vi "WPI_CameraSend Images To PC Loop.vi"(8 "error in (no error)":errorcluster, 9 "port":u16=1181) -> ()   [LabVIEW 2017]
doc: "This VI is used to serve images from one or more named cameras on your robot to the dashboard, SmartDashboard, or compatible web browser. Camera name and type info is published using network tables. Connections are on port 1181 by default and the URL for streaming can be found by looking at the network \"camera\"/streams variable. Cameras that are opened and stored in the name registry are automatically published by that name.\n\nThis VI runs in parallel with other code and should be placed in Robot Main or in Periodic Tasks.\n\nThis software is licensed. Open the labview\\readme\\WPI Robotics Library Open Source License.txt file for more information."
uses:
  <vilib>/Rock Robotics/WPI/Utilities/Refnum Registry Operation.ctl
  <vilib>/Rock Robotics/Network Tables/NT Write String Array.vi
  <vilib>/Rock Robotics/Network Tables/NT Write String.vi
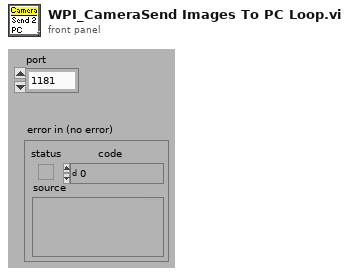
[diagram p1: front panel]
types:
  T1 = enum16{"Standard", "Buffered", "CRLF", "Immediate"}
  T2 = typedef "Refnum Registry Operation.ctl" = enum16{"set", "get", "delete", "get all names", "read name"}
  T3 = cluster{"token string":string, "token string 2":string}[]
  T4 = typedef "WPI_CameraDevRef.ctl" = cluster{"Camera Address":string, "CameraStatus":errorcluster}
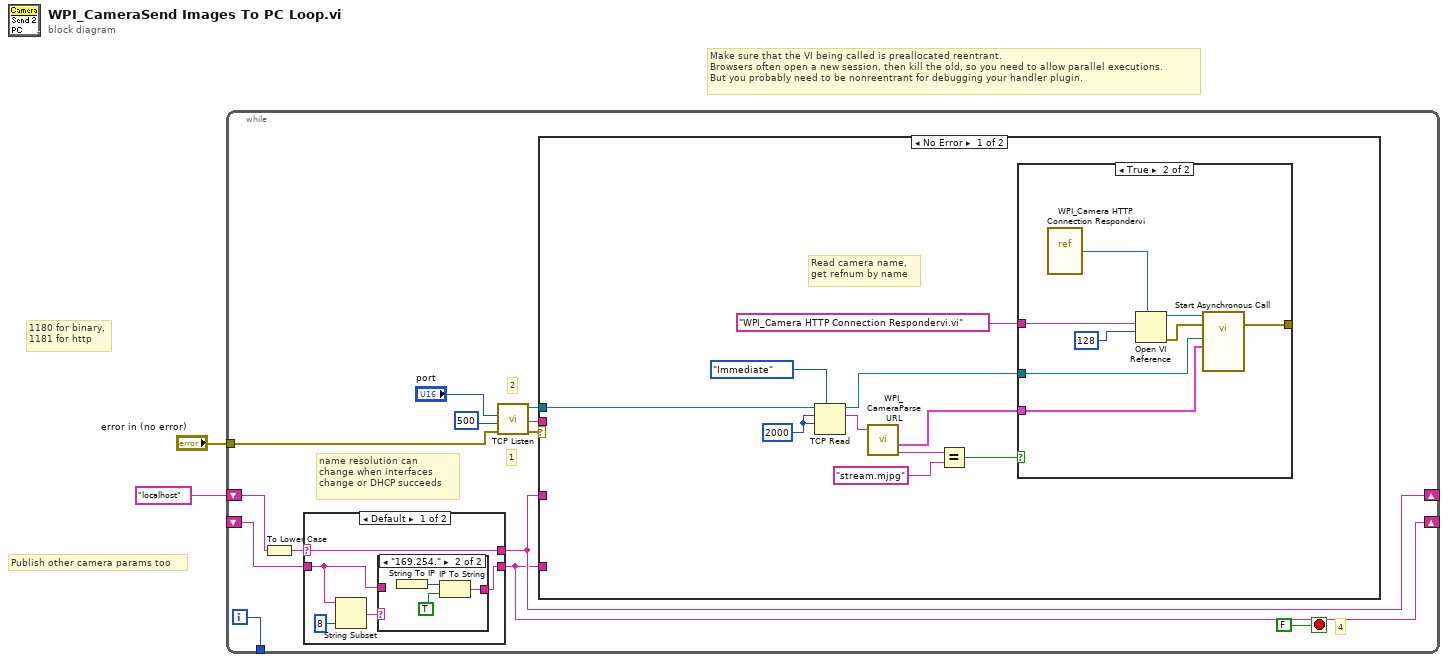
[diagram p0: block diagram]
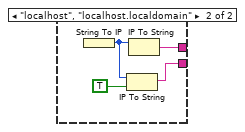
[diagram p3: hidden frame]
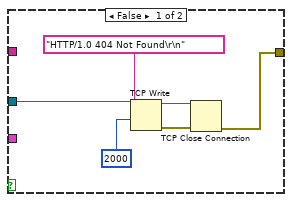
[diagram p4: hidden frame]
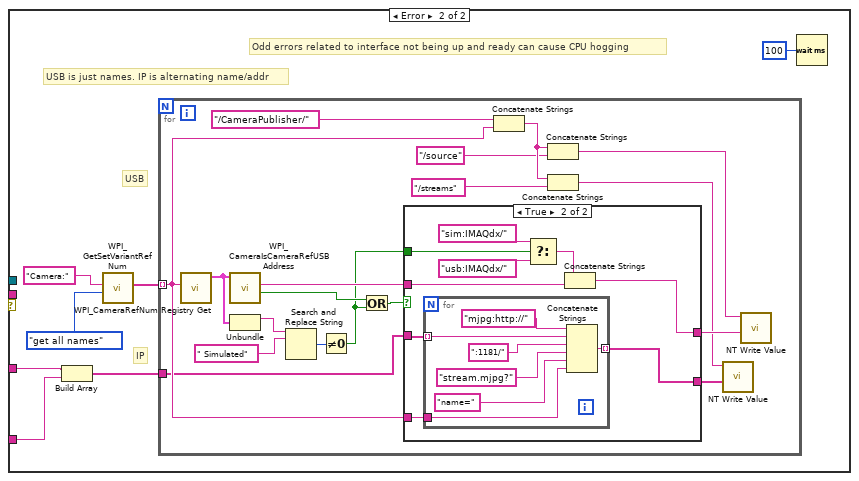
[diagram p5: hidden frame]
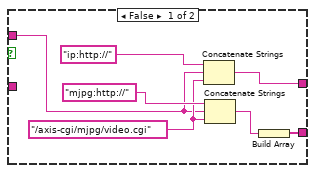
[diagram p6: hidden frame]
diagram:
  # "Make sure that the VI being called is preallocated reentrant.\nBrowsers often open a new session, then kill the old, so you need to allow parallel executions.\nBut you probably need to be nonreentrant for debugging your handler plugin."
  # "Publish other camera params too"
  # "1180 for binary,\n1181 for http"
  n1 = while {
    tunnel: "error in (no error)" -> [w14]
    tunnel: [w9] -> _
    shift-right: [w5] -> _
    shift-left: "localhost" -> [w6]
    shift-right: [w3] -> _
    shift-left: _ -> [w4]
    i -> [w9]
    stop <- FALSE ("status") stop-if-true
    # "name resolution can\nchange when interfaces\nchange or DHCP succeeds"
    # "4"
    # "1"
    # "2"
    n2 = To Lower Case(string=w6) -> (all lower case string=w7:string)
    n3 = case shown="Default" w7 {
      selector: w7 -> [w20 _]
      tunnel: [w20 w28] -> w5
      tunnel: w4 -> [w17 _]
      tunnel: [w16 w25] -> w3
      frame Default {
        n4 = String Subset(string=w17, length (rest)=8 ("length (rest)")) -> (substring=w18:string)  [unwired: 1 in]
        n5 = case shown="\"169.254.\"" w18 {
          tunnel: w17 -> [w21 _]
          tunnel: [w21 w22] -> w16
          frame Default {
          }
          frame "169.254." {
            n6 = String To IP() -> (0:w24:u32)  [unwired: 1 in]
            n7 = IP To String(1:TRUE ("dot notation? (F)"), 2:w24) -> (0:w22:string)
          }
        }
      }
      frame "localhost", "localhost.localdomain" {
        n8 = String To IP() -> (0:w26:u32)  [unwired: 1 in]
        n9 = IP To String(1:TRUE ("dot notation? (F)"), 2:w26) -> (0:w25:string)
        n10 = IP To String(2:w26) -> (0:w28:string)  [unwired: 1 in]
      }
    }
    n11 = call <vilib>:"TCP Listen.vi"("error in (no error)"=w14, "timeout ms (wait forever: -1)"=u16 500 ("port"), "port"="port") -> ("error out"=w11:errorcluster, "remote address"=w15:string, "connection ID"=w13:refnum<k5>)  [unwired: 1 in, 5 out]
    n12 = case shown="No Error" w11 {
      tunnel: w15 -> [_ _]
      tunnel: w13 -> [w35 _]
      tunnel: w5 -> [_ w55]
      tunnel: w3 -> [_ w53]
      frame No Error {
        w36 = 2000
        # "Read camera name,\nget refnum by name"
        n13 = TCP Read(connection ID=w35, bytes to read=w36, 7:T1."Immediate" ("mode (standard)"), 9:w36) -> (connection ID out=w34:refnum<k5>, data out=w29:string)  [unwired: 1 in, 1 out]
        n14 = call <vilib>:"WPI_CameraParse URL.vi"("URL"=w29) -> ("cgi string"=w31:string, "parameters"=w30:T3)  [unwired: 7 in, 2 out]
        n15 = Equal?(x=w31, y="stream.mjpg") -> (x = y?=w33:bool)
        n16 = case shown="True" w33 {
          tunnel: "WPI_Camera HTTP Connection Respondervi.vi" -> [_ w52]
          tunnel: w34 -> [w44 w48]
          tunnel: [w39 w46] -> _
          tunnel: w30 -> [_ w45]
          frame False {
            n17 = TCP Write(connection ID=w44, data in="HTTP/1.0 404 Not Found\r\n" ("regular expression"), 9:2000) -> (connection ID out=w43:refnum<k5>, error out=w40:errorcluster)  [unwired: 1 in, 1 out]
            n18 = TCP Close Connection(connection ID=w43, error in (no error)=w40) -> (error out=w39:errorcluster)  [unwired: 2 out]
          }
          frame True {
            n19 = vi-ref <vilib>:"WPI_Camera HTTP Connection Respondervi.vi"() -> (w50:refnum<vi>)
            n20 = Open VI Reference(type specifier VI Refnum (for type only)=w50, vi path=w52, options=128) -> (vi reference=w49:refnum<vi>, error out=w47:errorcluster)  [unwired: 3 in]
            n21 = call-by-ref "Start Asynchronous Call"(reference=w49, error in=w47, "parameters"=w45, "connection ID"=w48) -> (error out=w46:errorcluster)  [unwired: 10 in, 1 out]
          }
        }
      }
      frame Error {
        # "USB is just names. IP is alternating name/addr"
        # "IP"
        # "USB"
        # "Odd errors related to interface not being up and ready can cause CPU hogging"
        n22 = Build Array(w55, w53) -> (w54:string[])
        n23 = call <vilib>:"WPI_GetSetVariantRefNum.vi"("Operation"=Refnum_Registry_Operation."get all names" ("menu"), "refnum name"="Camera:") -> ("names"=w56:string[])  [unwired: 7 in, 2 out]
        n24 = for {
          tunnel: w56 -> [w75] mode=indexing
          tunnel: w54 -> [w60]
          n25 = call <vilib>:"WPI_CameraRefNum Registry Get.vi"("refnum name"=w75) -> ("CameraDevRef"=w66:T4)  [unwired: 9 in, 1 out]
          n26 = call <vilib>:"WPI_CameraIsCameraRefUSBAddress.vi"("CameraDevRef"=w66) -> ("USB?"=w63:bool, "Camera Address Out"=w68:string)  [unwired: 7 in, 2 out]
          n27 = Unbundle(w66) -> ("Camera Address"=w65:string)  [unwired: 1 out]
          n28 = Search and Replace String(input string=w65, search string=" Simulated") -> (number of replacements=w64:i32)  [unwired: 6 in, 3 out]
          n29 = Not Equal To 0?(x=w64) -> (x != 0?=w61:bool)
          n30 = Or(x=w63, y=w61) -> (x .or. y?=w62:bool)
          n31 = case shown="True" w62 {
            tunnel: w68 -> [w80 w91]
            tunnel: w60 -> [_ w93]
            tunnel: w75 -> [_ w92]
            tunnel: [w78 w90] -> w77
            tunnel: [w82 w85] -> w69
            tunnel: w61 -> [_ w89]
            frame False {
              w81 = "/axis-cgi/mjpg/video.cgi"
              n32 = Concatenate Strings("ip:http://", w80, w81) -> (w78:string)
              n33 = Concatenate Strings("mjpg:http://", w80, w81) -> (w83:string)
              n34 = Build Array(w83) -> (w82:string[])
            }
            frame True {
              n35 = for {
                tunnel: w93 -> [w99] mode=indexing
                tunnel: w92 -> [w95]
                tunnel: [w94] -> w85 mode=indexing
                n36 = Concatenate Strings("mjpg:http://", w99, ":1181/", "stream.mjpg?", "name=", w95) -> (w94:string)
              }
              n37 = Select(t="sim:IMAQdx/", s=w89, f="usb:IMAQdx/") -> (s? t:f=w86:string)
              n38 = Concatenate Strings(w86, w91) -> (w90:string)
            }
          }
          n39 = Concatenate Strings("/CameraPublisher/", w75) -> (w73:string)
          n40 = Concatenate Strings(w73, "/source") -> (w70:string)
          n41 = Concatenate Strings(w73, "/streams") -> (w71:string)
          n42 = call-poly <vilib>:"NT Write Value.vi"("String Array"=w69, "Name"=w71) -> ()  [unwired: 9 in, 1 out]
          n43 = call-poly <vilib>:"NT Write Value.vi"("String"=w77, "Name"=w70) -> ()  [unwired: 9 in, 1 out]
        }
        n44 = Wait (ms)(milliseconds to wait=u32 100) -> ()  [unwired: 1 out]
      }
    }
  }
